vi "Copy All (No Check).vi"(8 "error in (no error)":errorcluster, 10 "dst Pointer in":refnum<class "Pointer.lvclass">, 11 "src Pointer in":refnum<class "Pointer.lvclass">) -> (0 "error out":errorcluster, 2 "dst Pointer out":refnum<class "Pointer.lvclass">, 3 "src Pointer out":refnum<class "Pointer.lvclass">)   [LabVIEW 2017, in "Memory Manager.lvlib" / "Pointer.lvclass"]
doc: "Copies all of the data from the memory address specified by <b>src pointer</b> to the memory address specified by <b>dst pointer</b>.\n\n<b>Note:</b> This VI is <b>unsafe</b>.\n\nUnsafe means that this function does not have a check to ensure that the size of the source memory is inbounds of allocated memory for the destination before peforming a memory read/write. Reading/writing more data to a pointer than it has allocated can corrupt or crash LabVIEW. Only use this VI in scenarios where the <b>dst pointer</b> has been validated to be allocated to a correct size before calling this VI."
uses:
  Pointer.lvclass
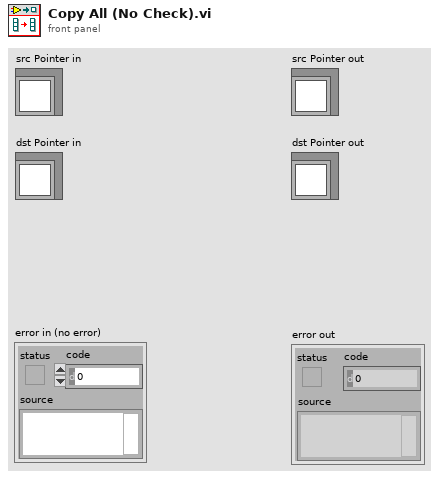
[diagram p1: front panel]
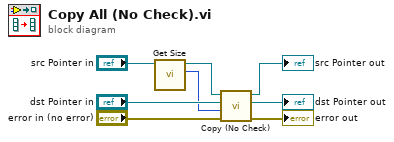
[diagram p0: block diagram]
diagram:
  n1 = call "Get Size.vi"("Pointer in"="src Pointer in") -> ("size"=w1:u64, "Pointer out"=w5:refnum<class "Pointer.lvclass">)  [unwired: 9 in]
  n2 = call "Copy (No Check).vi"("error in (no error)"="error in (no error)", "bytes to copy"=w1, "dst Pointer in"="dst Pointer in", "src Pointer in"=w5) -> ("error out"=→"error out":errorcluster, "dst Pointer out"=→"dst Pointer out":refnum<class "Pointer.lvclass">, "src Pointer out"=→"src Pointer out":refnum<class "Pointer.lvclass">)  [unwired: 4 in, 1 out]
